vi "contains_item.vi"(8 "error in (no error)":errorcluster, 10 "key_name":string, 11 "Table in":refnum<class "InlineTable.lvclass">) -> (0 "error out":errorcluster, 1 "contains_item":bool, 3 "Table out":refnum<class "InlineTable.lvclass">)   [LabVIEW 2020, in "toml_edit.lvlib" / "InlineTable.lvclass"]
uses:
  InlineTable.lvclass
  InlineTable.lvclass/InlineTable.ctl
  dragon_toml_32.dll
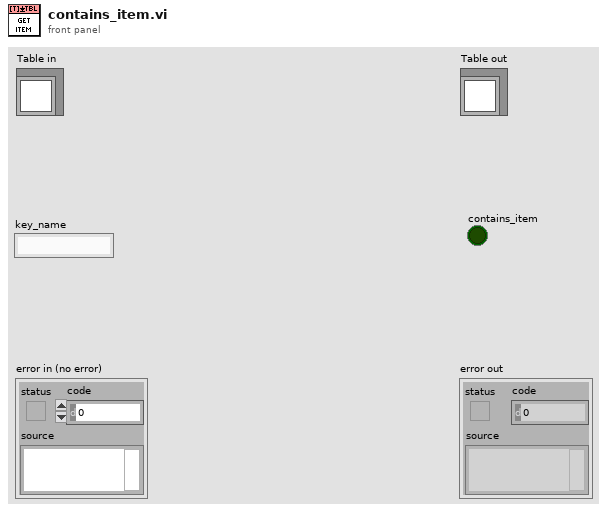
[diagram p1: front panel]
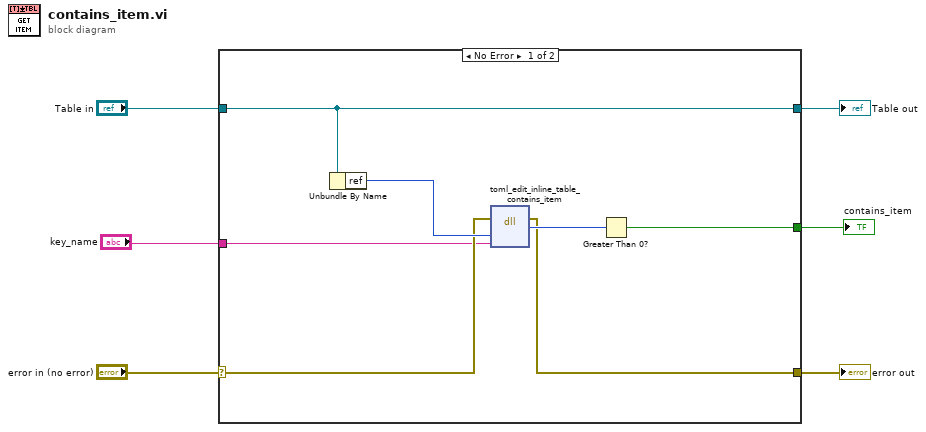
[diagram p0: block diagram]
diagram:
  n1 = case shown="No Error" "error in (no error)" {
    selector: "error in (no error)" -> [w10 w15]
    tunnel: [w9 w15] -> w5
    tunnel: [w13 w14] -> w3
    tunnel: "Table in" -> [w13 w14]
    tunnel: "key_name" -> [w7 _]
    tunnel: [w8 _] -> w1
    frame No Error {
      n2 = Unbundle By Name(w13) -> ("ref"=w11:u64)
      n3 = dll-call lib="C:/projects/dragon-desktop/source/submodules/toml-edit-labview/lv_src/dragon_toml_*.dll" fn="toml_edit_inline_table_contains_item"(error in=w10, "table_ref"=w11, "item_name"=w7) -> (error out=w9:errorcluster, "contains_item_bool"=w12:u64)  [unwired: 4 in, 1 out]
      n4 = Greater Than 0?(x=w12) -> (x > 0?=w8:bool)
    }
    frame Error {
    }
  }
  "error out" <- w5
  "Table out" <- w3
  "contains_item" <- w1
